vi "Scripting Constants.vi"() -> ()   [LabVIEW 2017, in "Routing and Faulting Scripting.lvlib"]
doc: "Use this Global VI to access the GUIDs assigned to the page resources of the Custom Device."
uses:
  Routing and Faulting Scripting.lvlib
panel:
  in  "Tab Control":enum32{"RaF Constants", "Properties", "GUID"}(tab)=enum."Properties"
  in  "RAF:Revisions:FQN":string="user.CD.Revisions"
  in  "RAF:Modules:FQN":string="user.CD.Modules"
  in  "RAF:Channel:Descriptions":string="Descriptions"
  in  "RAF:State:Description":string="_Description"
  in  "RAF:State:DefaultValue":i32
  in  "RAF:State:DefaultName":string="Default"
  in  "RAF:Channel:Connections":string="Connections"
  in  "Compiled.Settings":string="Compiled.Settings"
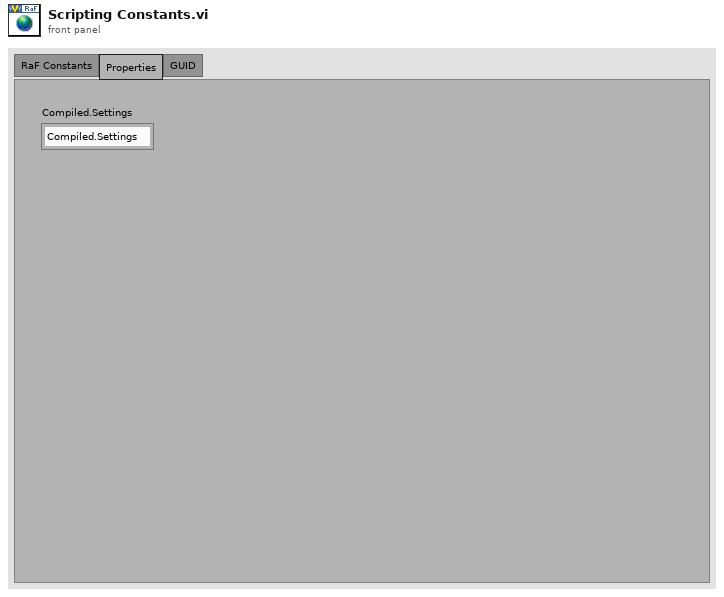
[diagram p1: front panel]
diagram:
